vi "Operation Main.vi"(8 "error in (no error)":errorcluster, 11 "Device Connector in":refnum<class "Device Connector.lvclass">) -> (0 "error out":errorcluster, 3 "Device Connector out":refnum<class "Device Connector.lvclass">)   [LabVIEW 2024, in "Device Connector.lvclass"]
uses:
  Device Connector.lvclass
  Device Connector MSG/Device Connector MSG.lvclass
  Ancestor Class/Message/Message.lvclass/Message.ctl
  Device Connector.lvclass/Device Connector.ctl
  Device Connector MSG/Device Connector MSG.lvclass/Device Connector MSG.ctl
  Ancestor Class/Message/Public Data/Read General CMD.vi
  Device Connector MSG/Public Data/Read Device Connector CMD.vi
  Ancestor Class/Message/Public Data/Read CMD Type.vi
  Ancestor Class/Message/Message.lvclass
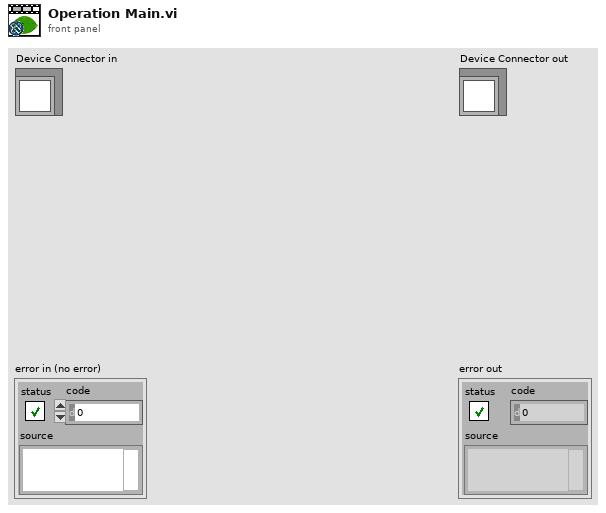
[diagram p1: front panel]
types:
  T1 = cluster{"Boolean Round":bool, "code":i32, "source":string}
  T2 = typedef "CMD Type.ctl" = enum16{"None", "General CMD", "1st CMD", "2nd CMD", "3rd CMD", "4th CMD", "5th CMD", "6th CMD", "7th CMD"}
  T3 = typedef "General CMD.ctl" = enum16{"None", "Stop", "Abort", "Running Task", "Running Batch Tasks", "Task Self Running", "Emergency Stop", "Subscribe", "UnSubscribe", "Pause", "Receive Parameters", "Active", "Resume"}
  T4 = typedef "Stop Observer Loop.ctl" = refnum<notifier>
  T5 = typedef "Device Connector CMD.ctl" = enum16{"None", "Subscribe Observer", "Cancel Subscribe", "Receive Request"}
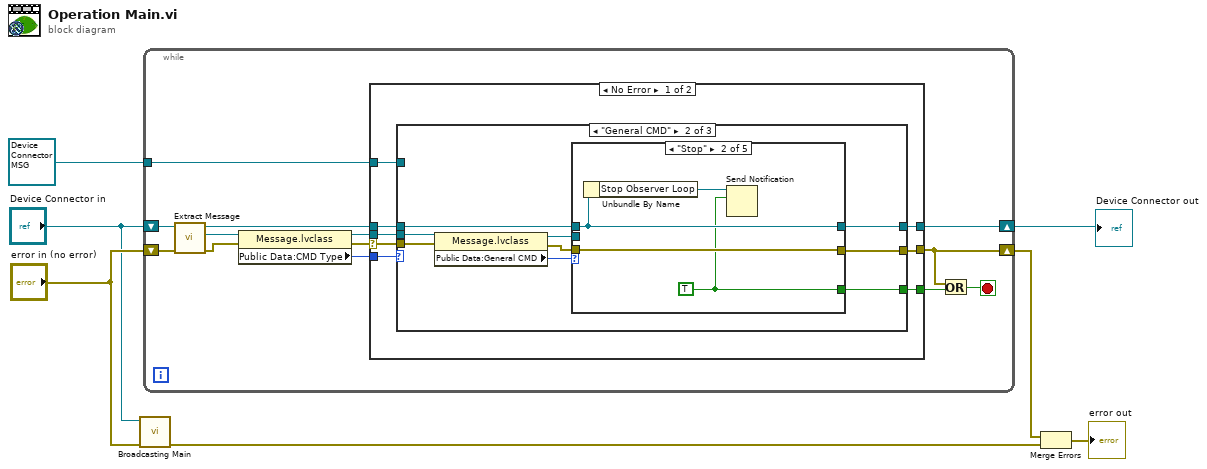
[diagram p0: block diagram]
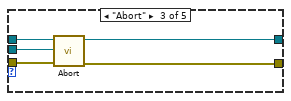
[diagram p4: hidden frame]
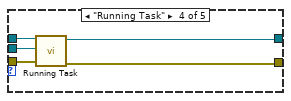
[diagram p5: hidden frame]
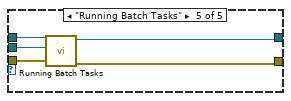
[diagram p6: hidden frame]
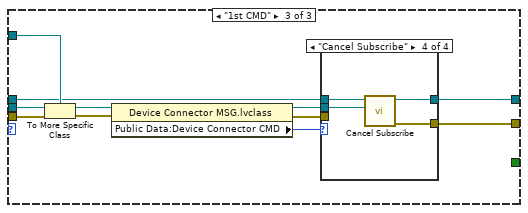
[diagram p7: hidden frame]
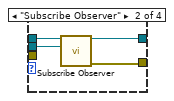
[diagram p9: hidden frame]
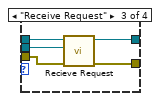
[diagram p10: hidden frame]
diagram:
  n1 = call "Broadcasting Main.vi"("Error In"="error in (no error)", "Device Connector in"="Device Connector in") -> ("error out (no error)"=w3:T1)  [unwired: 8 in, 1 out]
  n2 = while {
    shift-right: [w9] -> w7
    shift-left: "Device Connector in" -> [w14]
    shift-right: [w16] -> w2
    shift-left: "error in (no error)" -> [w13]
    tunnel: refnum<class "Device Connector MSG.lvclass"> refnum ("Device Connector MSG.lvclass") -> [w15]
    stop <- w17 stop-if-true
    n3 = call-dynamic "Extract Message.vi"("error in (no error)"=w13, "System Actor in"=w14) -> ("error out"=w10:errorcluster, "Message Out"=w11:refnum<class "Message.lvclass">, "System Actor out"=w12:refnum<class "Device Connector.lvclass">)  [unwired: 6 in, 1 out]
    n4 = property class="Message.lvclass"(reference=w11, error in=w10) -> (reference out=w18:refnum<class "Message.lvclass">, error out=w19:errorcluster, "Public Data:CMD Type"=w20:T2)
    n5 = case shown="No Error" w19 {
      selector: w19 -> [w24 w87]
      tunnel: w20 -> [w28 _]
      tunnel: w12 -> [w26 w88]
      tunnel: [w25 w88] -> w9
      tunnel: w18 -> [w27 _]
      tunnel: [w22 w87] -> w16
      tunnel: w15 -> [w23 _]
      tunnel: [w21 _] -> w8
      frame No Error {
        n6 = case shown="\"General CMD\"" w28 {
          tunnel: w27 -> [_ w39 w71]
          tunnel: w26 -> [w30 w36 w63]
          tunnel: [w30 w33 w62] -> w25
          tunnel: w24 -> [w29 w38 w70]
          tunnel: w23 -> [_ _ w69]
          tunnel: [w29 w32 w61] -> w22
          tunnel: [_ w31 _] -> w21
          frame "None", Default {
          }
          frame "General CMD" {
            n7 = property class="Message.lvclass"(reference=w39, error in=w38) -> (reference out=w35:refnum<class "Message.lvclass">, error out=w34:errorcluster, "Public Data:General CMD"=w37:T3)
            n8 = case shown="\"Stop\"" w37 {
              tunnel: w36 -> [w41 w44 w50 w55 w60]
              tunnel: w35 -> [_ _ w49 w53 w59]
              tunnel: w34 -> [w40 w45 w48 w52 w58]
              tunnel: [w41 w44 w47 w54 w57] -> w33
              tunnel: [w40 w45 w46 w51 w56] -> w32
              tunnel: [_ w42 _ _ _] -> w31
              frame "None", Default {
              }
              frame "Stop" {
                w42 = TRUE
                n9 = Unbundle By Name(w44) -> ("Stop Observer Loop"=w43:T4)
                n10 = Send Notification(notification=w42, notifier=w43) -> ()  [unwired: 1 in, 2 out]
              }
              frame "Abort" {
                n11 = call-dynamic "Abort.vi"("error in (no error)"=w48, "Message In"=w49, "System Actor in"=w50) -> ("error out"=w46:errorcluster, "System Actor out"=w47:refnum<class "Device Connector.lvclass">)  [unwired: 7 in]
              }
              frame "Running Task" {
                n12 = call-dynamic "Running Task.vi"("error in (no error)"=w52, "Message In"=w53, "System Actor in"=w55) -> ("error out"=w51:errorcluster, "System Actor out"=w54:refnum<class "Device Connector.lvclass">)  [unwired: 7 in]
              }
              frame "Running Batch Tasks" {
                n13 = call-dynamic "Running Batch Tasks.vi"("error in (no error)"=w58, "Message In"=w59, "System Actor in"=w60) -> ("error out"=w56:errorcluster, "System Actor out"=w57:refnum<class "Device Connector.lvclass">)  [unwired: 7 in]
              }
            }
          }
          frame "1st CMD" {
            n14 = To More Specific Class(target class=w69, reference=w71, error in=w70) -> (specific class reference=w68:refnum<class "Device Connector MSG.lvclass">, error out=w67:errorcluster)
            n15 = property class="Device Connector MSG.lvclass"(reference=w68, error in=w67) -> (reference out=w65:refnum<class "Device Connector MSG.lvclass">, error out=w64:errorcluster, "Public Data:Device Connector CMD"=w66:T5)
            n16 = case shown="\"Cancel Subscribe\"" w66 {
              tunnel: w65 -> [_ w76 w81 w85]
              tunnel: w64 -> [w72 _ w78 _]
              tunnel: w63 -> [w73 w77 w82 w86]
              tunnel: [w73 w75 w80 w84] -> w62
              tunnel: [w72 w74 w79 w83] -> w61
              frame "None", Default {
              }
              frame "Subscribe Observer" {
                n17 = call-dynamic "Subscribe Observer.vi"("Device Connector MSG In"=w76, "Device Connector in"=w77) -> ("error out"=w74:errorcluster, "Device Connector out"=w75:refnum<class "Device Connector.lvclass">)  [unwired: 8 in]
              }
              frame "Receive Request" {
                n18 = call-dynamic "Recieve Request.vi"("error in (no error)"=w78, "Device Connector MSG In"=w81, "Device Connector in"=w82) -> ("error out"=w79:errorcluster, "Device Connector out"=w80:refnum<class "Device Connector.lvclass">)  [unwired: 7 in]
              }
              frame "Cancel Subscribe" {
                n19 = call-dynamic "Cancel Subscribe.vi"("Device Connector MSG in"=w85, "Device Connector in"=w86) -> ("error out"=w83:errorcluster, "Device Connector out"=w84:refnum<class "Device Connector.lvclass">)  [unwired: 8 in]
              }
            }
          }
        }
      }
      frame Error {
      }
    }
    n20 = Or(x=w16, y=w8) -> (x .or. y?=w17:bool)
  }
  "Device Connector out" <- w7
  n21 = Merge Errors(w2, w3) -> (→"error out":errorcluster)
